vi "get project name.vi"(8 "error in":errorcluster) -> (0 "error out":errorcluster, 3 "Project name":string)   [LabVIEW 2020, in "Publisher Subscriber.lvlib"]
uses:
  Publisher Subscriber.lvlib
panel:
  # "This VI needs to be called from a project\nelse will throw the error"
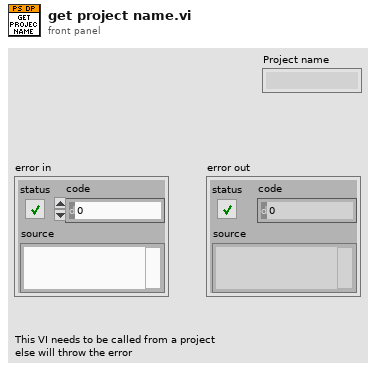
[diagram p1: front panel]
types:
  T1 = enum32{"invalid app kind", "Development System", "Run Time System", "Student Edition", "Embedded LabVIEW", "Evaluation", "Custom"}
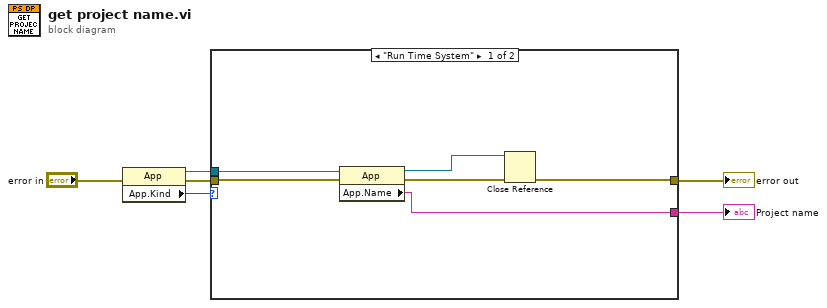
[diagram p0: block diagram]
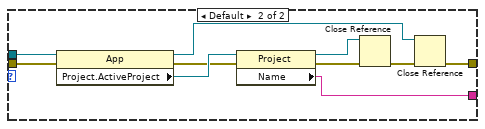
[diagram p2: hidden frame]
diagram:
  n1 = property class="App"(error in="error in") -> (reference out=w1:refnum<vi>, error out=w2:errorcluster, "App.Kind"=w4:T1)  [unwired: 1 in]
  n2 = case shown="\"Run Time System\"" w4 {
    tunnel: [w9 w22] -> w6
    tunnel: [w8 w21] -> w5
    tunnel: w2 -> [w10 w20]
    tunnel: w1 -> [w7 w13]
    frame "Run Time System" {
      n3 = property class="App"(reference=w7, error in=w10) -> (reference out=w12:refnum<vi>, error out=w11:errorcluster, "App.Name"=w8:string)
      n4 = Close Reference(reference=w12, error in (no error)=w11) -> (error out=w9:errorcluster)
    }
    frame Default {
      n5 = property class="App"(reference=w13, error in=w20) -> (reference out=w14:refnum<vi>, error out=w18:errorcluster, "Project.ActiveProject"=w19:refnum<vi>)
      n6 = property class="Project"(reference=w19, error in=w18) -> (reference out=w15:refnum<vi>, error out=w17:errorcluster, "Name"=w21:string)
      n7 = Close Reference(reference=w15, error in (no error)=w17) -> (error out=w16:errorcluster)
      n8 = Close Reference(reference=w14, error in (no error)=w16) -> (error out=w22:errorcluster)
    }
  }
  "error out" <- w6
  "Project name" <- w5
